vi "AlgorithmASolenoidAngleandPosition.vi"(2 "Theta in degrees":dbl, 3 "MartchBall Y":dbl) -> (0 "Ymovement":dbl, 1 "X movefromcenter":dbl)   [LabVIEW 2014]
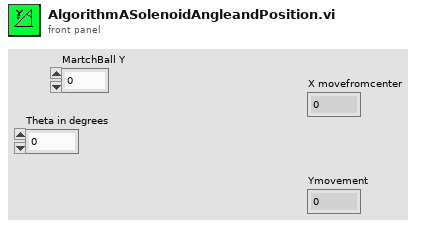
[diagram p1: front panel]
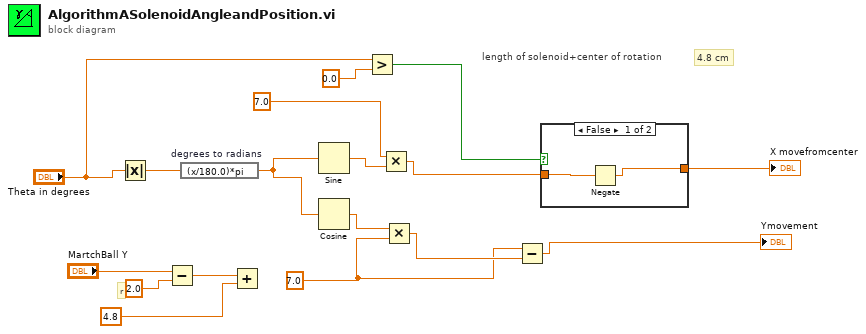
[diagram p0: block diagram]
diagram:
  w2 = 7.0
  # "r"
  # "4.8 cm"
  # "length of solenoid+center of rotation"
  n1 = Absolute Value(x="Theta in degrees") -> (abs(x)=w16:dbl)
  n2 = Subtract(x="MartchBall Y", y=2.0) -> (x-y=w5:dbl)
  n3 = expression code="(x/180.0)*pi" "degrees to radians"(w16) -> (w17:dbl)
  n4 = Add(x=w5, y=4.8) -> ()  [unwired: 1 out]
  n5 = Sine(x=w17) -> (sin(x)=w14:dbl)
  n6 = Cosine(x=w17) -> (cos(x)=w15:dbl)
  n7 = Greater?(x="Theta in degrees", y=0.0) -> (0:w13:bool)
  n8 = Multiply(x=7.0, y=w14) -> (x*y=w10:dbl)
  n9 = Multiply(x=w15, y=w2) -> (x*y=w8:dbl)
  n10 = Subtract(x=w2, y=w8) -> (x-y=→"Ymovement":dbl)
  n11 = case shown="False" w13 {
    tunnel: w10 -> [w18 w20]
    tunnel: [w19 w20] -> w9
    frame False {
      n12 = Negate(x=w18) -> (-x=w19:dbl)
    }
    frame True {
    }
  }
  "X movefromcenter" <- w9
